vi "Obs_air.vi"(4 "Reset_x":i32=800, 6 "Return_x":i32=-50, 7 "Mov_Spd":i32=5, 8 "error in":errorcluster, 10 "Obs A_Ref":refnum<vi>) -> (0 "error out":errorcluster, 2 "active":bool)   [LabVIEW 2012]
panel:
  # "橫跨畫面一次後deactive"
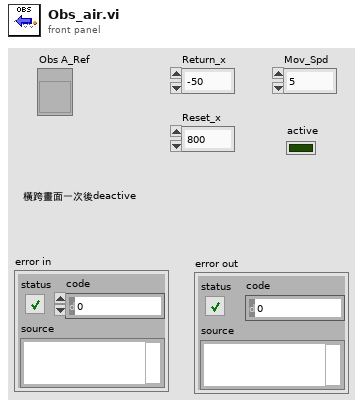
[diagram p1: front panel]
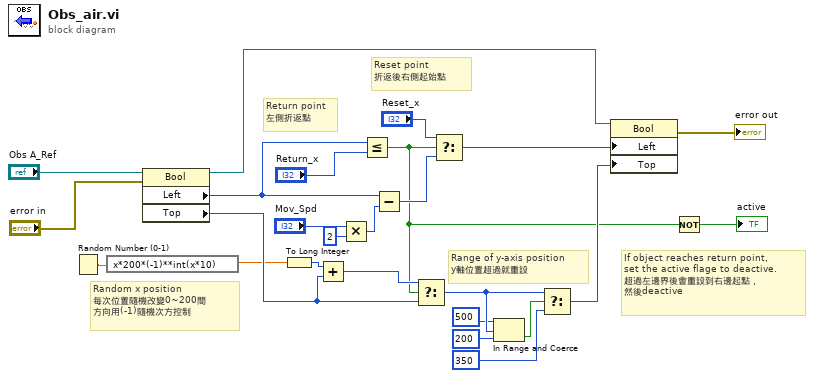
[diagram p0: block diagram]
diagram:
  # "If object reaches return point,\nset the active flage to deactive.\n超過左邊界後會重設到右邊起點，\n然後deactive"
  # "Range of y-axis position\ny軸位置超過就重設"
  # "Random x position\n每次位置隨機改變0~200間\n方向用(-1)隨機次方控制"
  # "Return point\n左側折返點"
  # "Reset point\n折返後右側起始點"
  n1 = Random Number (0-1)() -> (number: 0 to 1=w18:dbl)
  n2 = expression code="x*200*(-1)**int(x*10)"(w18) -> (w20:dbl)
  n3 = property on="Property Node" class="Bool"(reference="Obs A_Ref", error in="error in") -> (reference out=w15:refnum<vi>, "Left"=w23:i32, "Top"=w22:i32)  [unwired: 1 out]
  n4 = To Long Integer(number=w20) -> (32bit integer=w19:i32)
  n5 = Add(x=w19, y=w22) -> (x+y=w21:i32)
  n6 = Multiply(x="Mov_Spd", y=2) -> (x*y=w5:i32)
  n7 = Less Or Equal?(x=w23, y="Return_x") -> (x <= y?=w2:bool)
  n8 = Subtract(x=w23, y=w5) -> (x-y=w16:i32)
  n9 = Select(t=w21, s=w2, f=w22) -> (s? t:f=w11:i32)
  n10 = Select(t="Reset_x", s=w2, f=w16) -> (s? t:f=w25:i32)
  n11 = In Range and Coerce(upper limit=500 ("y"), x=w11, lower limit=200 ("y")) -> (In Range?=w14:bool)  [unwired: 1 out]
  n12 = Select(t=w11, s=w14, f=350 ("y")) -> (s? t:f=w12:i32)
  n13 = property on="Property Node" class="Bool"(reference=w15, "Left"=w25, "Top"=w12) -> (error out=→"error out":errorcluster)  [unwired: 1 in, 1 out]
  n14 = Not(x=w2) -> (.not. x?=→"active":bool)
